vi "tqhjinformation.vi"(0 "object in":refnum<class "212format_work.lvclass">, 1 "in":T1, 5 "error in (no error)":errorcluster) -> (14 "object out":refnum<class "212format_work.lvclass">, 15 "out":T2, 19 "error out":errorcluster)   [LabVIEW 2016, in "212format_work.lvclass"]
uses:
  212format_work.lvclass
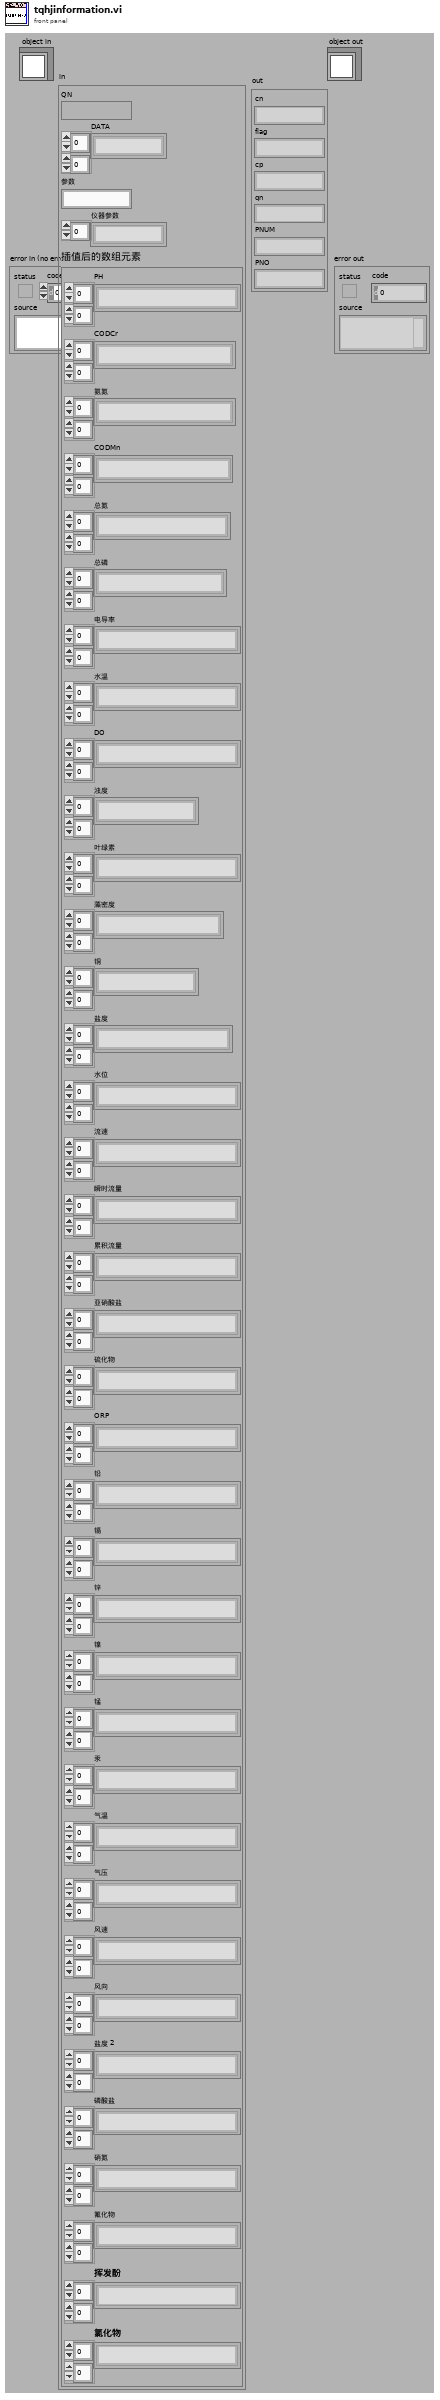
[diagram p1: front panel]
types:
  T1 = cluster{"QN":string, "DATA":string[][], "参数":string, "仪器参数":string[], "插值后的数组元素":cluster{"PH":string[][], "CODCr":string[][], "氨氮":string[][], "CODMn":string[][], "总氮":string[][], "总磷":string[][], "电导率":string[][], "水温":string[][], "DO":string[][], "浊度":string[][], "叶绿素":string[][], "藻密度":string[][], "铜":string[][], "盐度":string[][], "水位":string[][], "流速":string[][], "瞬时流量":string[][], "累积流量":string[][], "亚硝酸盐":string[][], "硫化物":string[][], "ORP":string[][], "铅":string[][], "镉":string[][], "锌":string[][], "镍":string[][], "锰":string[][], "汞":string[][], "气温":string[][], "气压":string[][], "风速":string[][], "风向":string[][], "盐度 2":string[][], "磷酸盐":string[][], "硝氮":string[][], "氟化物":string[][], "挥发酚":string[][], "氯化物":string[][]}}
  T2 = cluster{"cn":string, "flag":string, "cp":string, "qn":string, "PNUM":string, "PNO":string}
  T3 = typedef "212format_work.lvclass/interdata控件.ctl" = cluster{"数据发送协议":enum16{"2005-212协议", "2017-212协议"}, "枚举":enum16{"返回请求应答", "上传数据", "返回执行结果"}, "系统编码ST":string, "主动上报数据中":bool, "数据组合发送":bool, "地表水/污染源":bool, "应用环境":enum16{"STD", "GB212"}}
  T4 = typedef "212format_work.lvclass/data控件.ctl" = cluster{"选择发送的参数":string, "插值后的数组元素":cluster{"PH":string[][], "CODCr":string[][], "氨氮":string[][], "CODMn":string[][], "总氮":string[][], "总磷":string[][], "电导率":string[][], "水温":string[][], "DO":string[][], "浊度":string[][], "叶绿素":string[][], "藻密度":string[][], "铜":string[][], "盐度":string[][], "水位":string[][], "流速":string[][], "瞬时流量":string[][], "累积流量":string[][], "亚硝酸盐":string[][], "硫化物":string[][], "ORP":string[][], "铅":string[][], "镉":string[][], "锌":string[][], "镍":string[][], "锰":string[][], "汞":string[][], "气温":string[][], "气压":string[][], "风速":string[][], "风向":string[][], "盐度 2":string[][], "磷酸盐":string[][], "硝氮":string[][], "氟化物":string[][], "挥发酚":string[][], "氯化物":string[][]}, "register values":u16[], "columns输出":string[], "环境参数":string[][], "仪器编码":string, "实时数据发送间隔":u32, "实时数据参数":string, "参数系数簇":cluster{"CODMn":dbl, "CODCr":dbl, "DO":dbl, "铜":dbl, "PH":dbl, "氨氮":dbl, "比电导率":dbl, "水温":dbl, "COD":dbl, "浊度":dbl, "总氮":dbl, "总磷":dbl, "叶绿素a":dbl, "藻密度":dbl, "水位":dbl, "流速":dbl, "瞬时流量":dbl, "累积流量":dbl, "亚硝酸盐":dbl, "硫化物":dbl, "ORP":dbl, "铅":dbl, "镉":dbl, "锌":dbl, "镍":dbl, "锰":dbl, "汞":dbl, "气温":dbl, "气压":dbl, "风速":dbl, "风向":dbl, "盐度":dbl, "磷酸盐":dbl, "硝氮":dbl, "氟化物":dbl, "挥发酚":dbl, "氯化物":dbl}, "因子编码簇":cluster{"CODMn":string, "CODCr":string, "DO":string, "铜":string, "PH":string, "氨氮":string, "比电导率":string, "水温":string, "COD":string, "浊度":string, "总氮":string, "总磷":string, "叶绿素a":string, "藻密度":string, "水位":string, "流速":string, "瞬时流量":string, "累积流量":string, "亚硝酸盐":string, "硫化物":string, "ORP":string, "铅":string, "镉":string, "锌":string, "镍":string, "锰":string, "汞":string, "气温":string, "气压":string, "风速":string, "风向":string, "盐度":string, "磷酸盐":string, "硝氮":string, "氟化物":string, "挥发酚":string, "氯化物":string}, "小时数据发送次数":i32, "读取试剂余量的值":u16[], "参数编码":string, "数据数组大小":i32, "总包数":i32, "当前包号":i32, "columns":string[], "剖面多参数":string[][], "分包标准":i32}
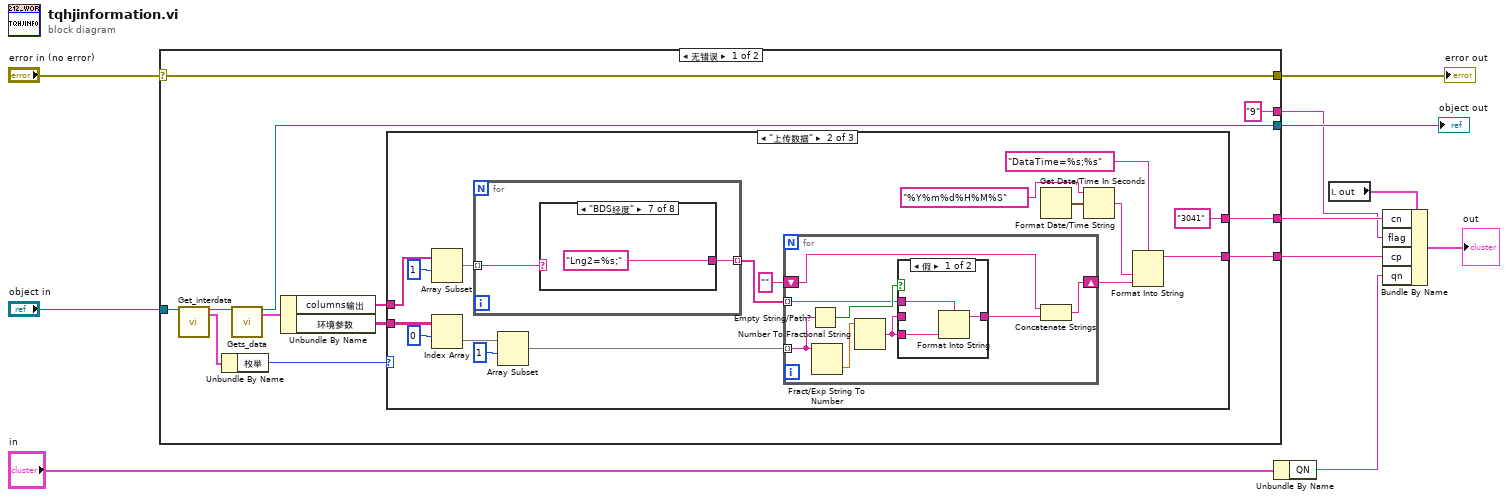
[diagram p0: block diagram]
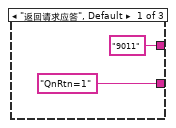
[diagram p2: hidden frame]
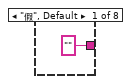
[diagram p3: hidden frame]
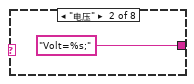
[diagram p4: hidden frame]
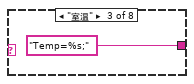
[diagram p5: hidden frame]
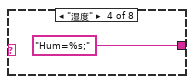
[diagram p6: hidden frame]
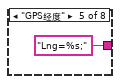
[diagram p7: hidden frame]
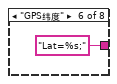
[diagram p8: hidden frame]
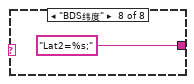
[diagram p9: hidden frame]
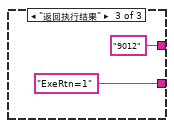
[diagram p11: hidden frame]
diagram:
  n1 = case shown="无错误" "error in (no error)" {
    selector: "error in (no error)" -> [w23 w68]
    tunnel: [w23 w68] -> w10
    tunnel: [w16 w67] -> w8
    tunnel: "object in" -> [w21 w67]
    tunnel: [w14 _] -> w3
    tunnel: [w18 _] -> w5
    tunnel: ["9" ("ST") _] -> w4
    frame No Error {
      n2 = call-dynamic "Get_interdata.vi"("object in"=w21) -> ("object out"=w17:refnum<class "212format_work.lvclass">, "interdata"=w20:T3)  [unwired: 16 in, 1 out]
      n3 = Unbundle By Name(w20) -> ("枚举"=w19:enum16{"返回请求应答", "上传数据", "返回执行结果"})
      n4 = call-dynamic "Gets_data.vi"("object in"=w17) -> ("object out"=w16:refnum<class "212format_work.lvclass">, "data"=w15:T4)  [unwired: 16 in, 1 out]
      n5 = Unbundle By Name(w15) -> ("columns输出"=w13:string[], "环境参数"=w12:string[][])
      n6 = case shown="\"上传数据\"" w19 {
        tunnel: ["9011" ("CN") "3041" ("CN") "9012" ("CN")] -> w18
        tunnel: ["QnRtn=1" w26 "ExeRtn=1"] -> w14
        tunnel: w13 -> [_ w27 _]
        tunnel: w12 -> [_ w28 _]
        frame "返回请求应答", Default {
        }
        frame "上传数据" {
          n7 = Array Subset(array=w27, index=1 ("索引")) -> (w34:string[])  [unwired: 1 in]
          n8 = Index Array(array=w28, index (row)=0 ("索引 (行)")) -> (element=w38:string[])  [unwired: 1 in]
          n9 = for {
            tunnel: w34 -> [w44] mode=indexing
            tunnel: [w43] -> w33 mode=indexing
            n10 = case shown="\"BDS经度\"" w44 {
              tunnel: ["" "Volt=%s;" "Temp=%s;" ("格式字符串") "Hum=%s;" ("格式字符串") "Lng=%s;" "Lat=%s;" "Lng2=%s;" "Lat2=%s;"] -> w43
              frame "假", Default {
              }
              frame "电压" {
              }
              frame "室温" {
              }
              frame "湿度" {
              }
              frame "GPS经度" {
              }
              frame "GPS纬度" {
              }
              frame "BDS经度" {
              }
              frame "BDS纬度" {
              }
            }
          }
          n11 = Array Subset(array=w38, index=1 ("索引")) -> (w36:string[])  [unwired: 1 in]
          n12 = for {
            shift-right: [w58] -> w41
            shift-left: "" -> [w57]
            tunnel: w33 -> [w56] mode=indexing
            tunnel: w36 -> [w54] mode=indexing
            n13 = Empty String/Path?(string/path=w54) -> (empty?=w60:bool)
            n14 = Fract/Exp String To Number(string=w54) -> (number=w55:dbl)  [unwired: 3 in, 1 out]
            n15 = Number To Fractional String(number=w55) -> (F-format string=w53:string)  [unwired: 3 in]
            n16 = case shown="假" w60 {
              tunnel: [w63 w64] -> w59
              tunnel: w56 -> [w62 _]
              tunnel: w53 -> [w61 _]
              tunnel: w53 -> [_ w64]
              frame False {
                n17 = Format Into String(format string=w62, w61) -> (resulting string=w63:string)  [unwired: 2 in, 1 out]
              }
              frame True {
              }
            }
            n18 = Concatenate Strings(w57, w59) -> (w58:string)
          }
          n19 = Get Date/Time In Seconds() -> (seconds since 1Jan1904=w31:timestamp)
          n20 = Format Date/Time String(time format string (%c)="%Y%m%d%H%M%S" ("时间格式字符串(%c)"), seconds (now)=w31) -> (date/time string=w32:string)  [unwired: 1 in]
          n21 = Format Into String(format string="DataTime=%s;%s" ("格式字符串"), w32, w41) -> (resulting string=w26:string)  [unwired: 2 in, 1 out]
        }
        frame "返回执行结果" {
        }
      }
    }
    frame Error {
    }
  }
  "error out" <- w10
  "object out" <- w8
  n22 = Unbundle By Name("in") -> ("QN"=w1:string)
  n23 = local read "out"() -> (w7:T2)
  n24 = Bundle By Name(cluster=w7, "cn"=w5, "flag"=w4, "cp"=w3, "qn"=w1) -> (→"out":T2)
